vi "PL_model.vi"(3 "output control":T1, 4 "data":variant, 5 "X":dbl[](array[numeric]), 6 "a":dbl[](array[numeric])) -> (0 "error out":errorcluster, 1 "f'(X,a)":dbl[][](array[numeric]), 2 "f(X,a)":dbl[](array[numeric]))   [LabVIEW 2018]
doc: "This template is the starting point for creating a model function to be passed to the Nonlinear Curve Fit.vi."
uses:
  <vilib>/gmath/NumericalOptimization/LM_output select.ctl
  <vilib>/gmath/NI_Gmath.lvlib
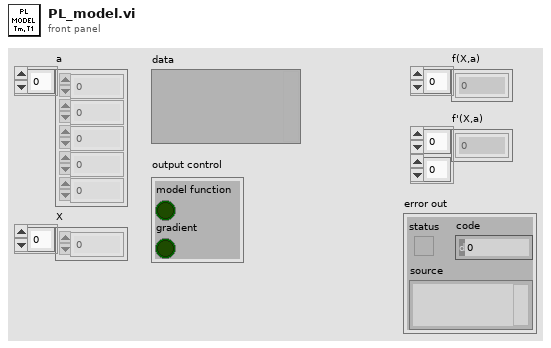
[diagram p1: front panel]
types:
  T1 = typedef "NI_Gmath.lvlib/LM_output select.ctl" = cluster{"model function":bool, "gradient":bool}
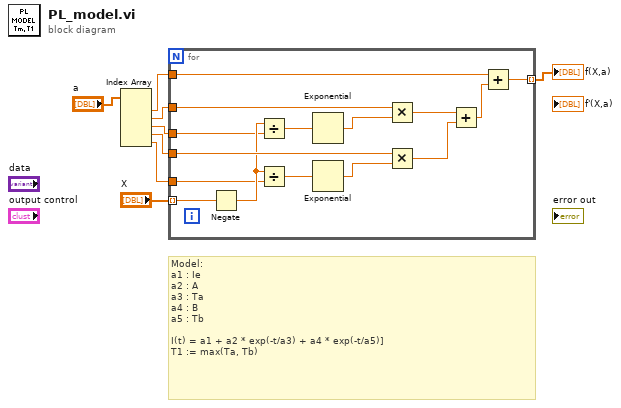
[diagram p0: block diagram]
diagram:
  # "Model:\na1 : Ie\na2 : A\na3 : Ta\na4 : B\na5 : Tb\n\nI(t) = a1 + a2 * exp(-t/a3) + a4 * exp(-t/a5)]\nT1 := max(Ta, Tb)"
  n1 = Index Array(array="a") -> (element #1=w1:dbl, element #2=w5:dbl, element #3=w4:dbl, element #4=w3:dbl, element #5=w2:dbl)  [unwired: 5 in]
  n2 = for {
    tunnel: w1 -> [w19]
    tunnel: w5 -> [w14]
    tunnel: w4 -> [w10]
    tunnel: w3 -> [w15]
    tunnel: w2 -> [w9]
    tunnel: [w18] -> w7 mode=indexing
    tunnel: "X" -> [w17] mode=indexing
    n3 = Negate(x=w17) -> (-x=w13:dbl)
    n4 = Divide(x=w13, y=w10) -> (x/y=w11:dbl)
    n5 = Divide(x=w13, y=w9) -> (x/y=w12:dbl)
    n6 = Exponential(1:w11) -> (0:w20:dbl)
    n7 = Exponential(1:w12) -> (0:w21:dbl)
    n8 = Multiply(x=w14, y=w20) -> (x*y=w16:dbl)
    n9 = Multiply(x=w15, y=w21) -> (x*y=w22:dbl)
    n10 = Add(x=w16, y=w22) -> (x+y=w23:dbl)
    n11 = Add(x=w19, y=w23) -> (x+y=w18:dbl)
  }
  "f(X,a)" <- w7
